vi "UMLEditor drawGrabbers.vi"(1 "graphics":refnum<class "Graphics.lvclass">, 2 "points":T1[](array[typedef]) {"y" format="%.2f"; "x" format="%.2f"}, 5 "error in (no error)":errorcluster) -> (19 "error out":errorcluster)   [LabVIEW 2012]
doc: "Draws grabbers"
uses:
  <resource>/Framework/Providers/Open_GDS/UML/General/Point/Point Point2D.ctl
  <resource>/Framework/Providers/Open_GDS/UML/Graphics_class/Graphics.lvclass
  <resource>/Framework/Providers/Open_GDS/UML/General/Rectangle/Rectangle Rectangle2D.ctl
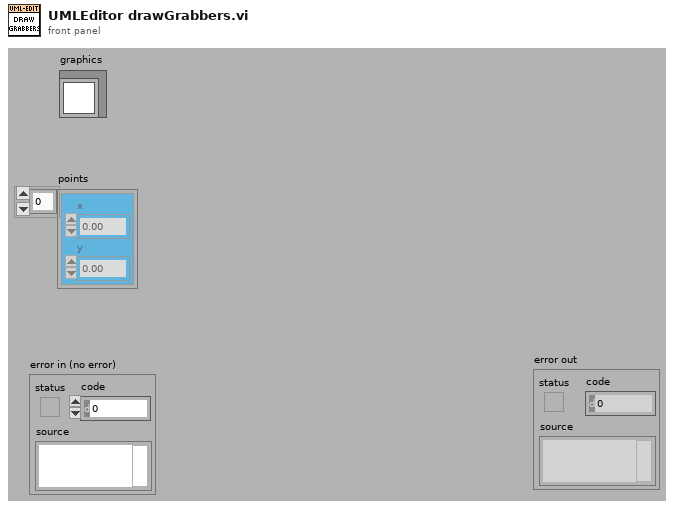
[diagram p1: front panel]
types:
  T1 = typedef "Point Point2D.ctl" = cluster{"x":dbl, "y":dbl}
  T2 = typedef "Rectangle Rectangle2D.ctl" = cluster{"x":dbl, "y":dbl, "width":dbl, "height":dbl}
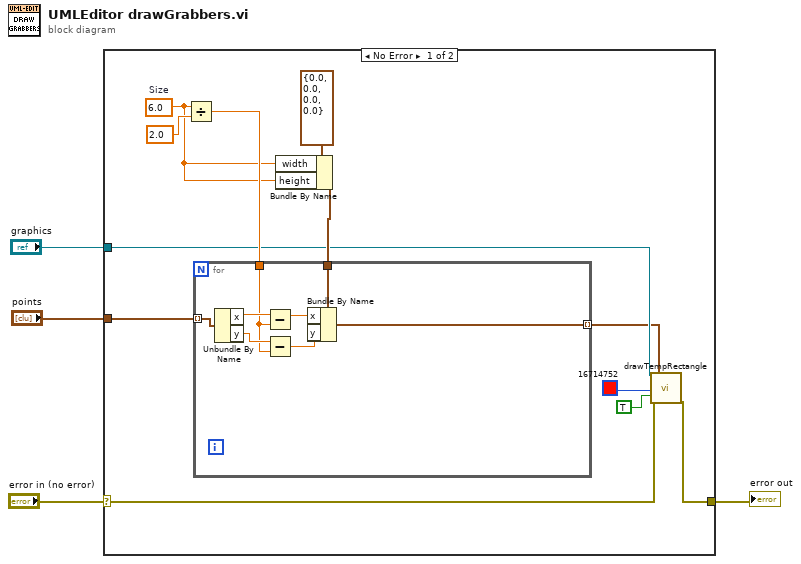
[diagram p0: block diagram]
diagram:
  n1 = case shown="No Error" "error in (no error)" {
    selector: "error in (no error)" -> [w6 w25]
    tunnel: [w5 w25] -> w3
    tunnel: "graphics" -> [w8 _]
    tunnel: "points" -> [w16 _]
    frame No Error {
      w12 = 6.0  # Size
      n2 = Divide(x=w12, y=2.0) -> (x/y=w14:dbl)
      n3 = Bundle By Name(cluster=T2 {"x"=0.0, "y"=0.0, "width"=0.0, "height"=0.0} ("rectangle"), "width"=w12, "height"=w12) -> (w11:T2)
      n4 = for {
        tunnel: w16 -> [w24] mode=indexing
        tunnel: w14 -> [w21]
        tunnel: w11 -> [w20]
        tunnel: [w17] -> w7 mode=indexing
        n5 = Unbundle By Name(w24) -> ("x"=w23:dbl, "y"=w22:dbl)
        n6 = Subtract(x=w23, y=w21) -> (x-y=w19:dbl)
        n7 = Subtract(x=w22, y=w21) -> (x-y=w18:dbl)
        n8 = Bundle By Name(cluster=w20, "x"=w19, "y"=w18) -> (w17:T2)
      }
      n9 = call <resource>:"drawTempRectangle.vi"("reference"=w8, "color(if not used=default color)"=u32 16714752, "fill?(F)"=TRUE, "error in (no error)"=w6, "Rectangles"=w7) -> ("error out"=w5:errorcluster)  [unwired: 3 in, 11 out]
    }
    frame Error {
    }
  }
  "error out" <- w3
